vi "FindPoint.vi"(9 "Vertical":i32, 10 "Horizontal":i32, 11 "Value":i32[][](array[numeric])) -> (3 "Numeric":i32)   [LabVIEW 2017]
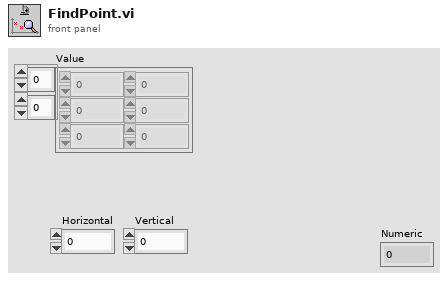
[diagram p1: front panel]
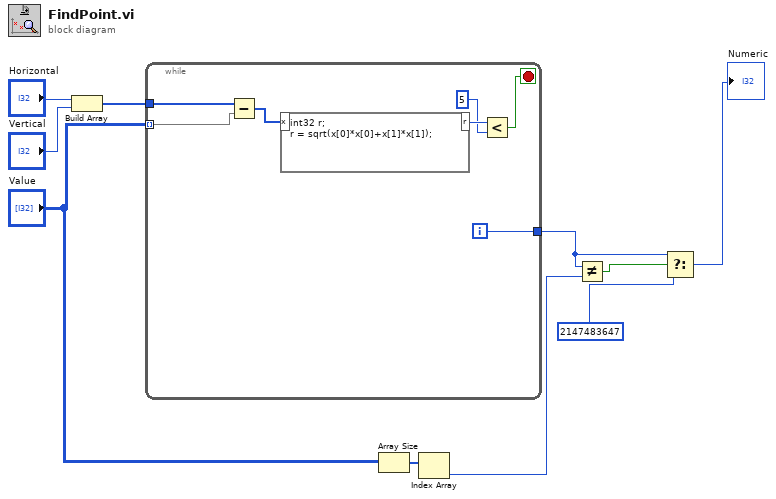
[diagram p0: block diagram]
diagram:
  n1 = Build Array("Horizontal", "Vertical") -> (w8:i32[])
  n2 = while {
    tunnel: "Value" -> [w17] mode=indexing
    tunnel: w8 -> [w16]
    tunnel: [w11] -> w4
    i -> [w11]
    stop <- w12 stop-if-true
    n3 = Subtract(x=w16, y=w17) -> (x-y=w15:i32[])
    n4 = formula code="int32 r;\nr = sqrt(x[0]*x[0]+x[1]*x[1]);"("x"=w15) -> ("r"=w14:i32)
    n5 = Less?(x=w14, y=5) -> (x < y?=w12:bool)
  }
  n6 = Array Size(array="Value") -> (size(s)=w6:i32[])
  n7 = Index Array(array=w6) -> (element=w2:i32)  [unwired: 1 in]
  n8 = Not Equal?(x=w4, y=w2) -> (x != y?=w3:bool)
  n9 = Select(t=w4, s=w3, f=2147483647) -> (s? t:f=→"Numeric":i32)
